vi "Running Voltmeter Average.vi"(2 "Point #":i32, 3 "Type":enum16{"DMM", "HP 34401", "Keithley 2001"}(ring), 4 "Instrument Address":refnum<visa-resource-name>) -> (0 "Stop":bool, 1 "?":dbl[](array[numeric]) format="%.4e")   [LabVIEW 2020]
doc: "This VI takes a running difference of 3 measurements of a HP34401 DMM. It assumes that the current has been reversed for the middle measurements. The value returned is the average of the 1st and 3rd measurements minus the 2nd measurement over 2.\nScott Hannahs, NHMFL - FSU, April 1995"
panel:
  out "Array":dbl[][][](array[numeric]) format="%.4e"
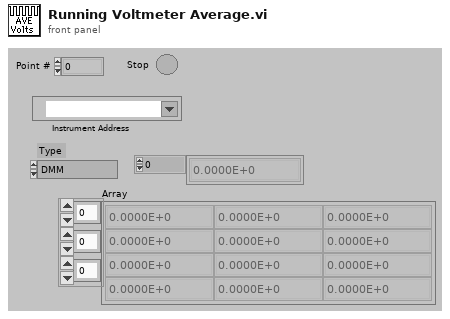
[diagram p1: front panel]
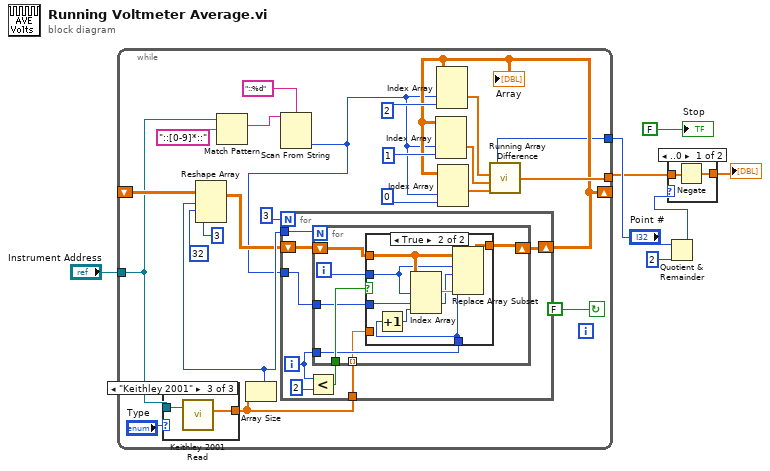
[diagram p0: block diagram]
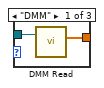
[diagram p2: hidden frame]
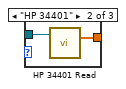
[diagram p3: hidden frame]
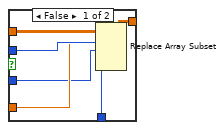
[diagram p4: hidden frame]
diagram:
  n1 = while {
    tunnel: "Point #" -> [w15]
    tunnel: "Instrument Address" -> [w8]
    tunnel: [w30] -> w4
    shift-left: _ -> [w19]
    shift-right: [w17] -> _
    stop <- FALSE continue-if-true
    n2 = case shown="\"Keithley 2001\"" "Type" {
      tunnel: w8 -> [w31 w34 w35]
      tunnel: [w32 w33 w36] -> w26
      frame "DMM" {
        n3 = call "DMM Read.vi"("Instrument Address"=w31) -> ("Measurement"=w32:dbl[])  [unwired: 1 in, 1 out]
      }
      frame "HP 34401" {
        n4 = call "HP 34401 Read.vi"("Instrument Address"=w34) -> ("Measurement"=w33:dbl[])  [unwired: 1 in, 1 out]
      }
      frame "Keithley 2001" {
        n5 = call "Keithley 2001 Read.vi"("Instrument Address"=w35) -> ("Measurement"=w36:dbl[])  [unwired: 1 in, 1 out]
      }
    }
    n6 = Match Pattern(string=w8, regular expression="::[0-9]*::") -> (match substring=w11:string)  [unwired: 1 in, 3 out]
    n7 = Array Size(array=w26) -> (size(s)=w25:i32)
    n8 = Reshape Array(w19, w25, 32, 3) -> (w18:dbl[][][])
    n9 = Scan From String(format string="::%d" ("Format String"), input string=w11) -> (output 1=w9:i32)  [unwired: 3 in, 3 out]
    n10 = for {
      N: 3 -> [_]
      tunnel: w9 -> [w39]
      tunnel: w26 -> [w44]
      tunnel: w25 -> [w40]
      shift-right: [w37] -> w17
      shift-left: w18 -> [w38]
      i -> [w43]
      n11 = Less?(x=w43, y=2) -> (x < y?=w41:bool)
      n12 = for {
        N: w40 -> [_]
        tunnel: w44 -> [w49] mode=indexing
        tunnel: w41 -> [w51]
        tunnel: w43 -> [w50]
        tunnel: w39 -> [w47]
        shift-right: [w45] -> w37
        shift-left: w38 -> [w46]
        i -> [w48]
        n13 = case shown="True" w51 {
          tunnel: w46 -> [w57 w59]
          tunnel: w50 -> [w56 w63]
          tunnel: [w55 w62] -> w45
          tunnel: w48 -> [w54 w58]
          tunnel: w49 -> [w53 _]
          tunnel: w47 -> [w52 w60]
          frame False {
            n14 = Replace Array Subset(array=w57, new element=w53, index (dim 0)=w54, index (dim 1)=w52, index (dim 2)=w56) -> (w55:dbl[][][])
          }
          frame True {
            n15 = Increment(x=w63) -> (x+1=w64:i32)
            n16 = Index Array(array=w59, index (dim 0)=w58, index (dim 1)=w60, index (dim 2)=w64) -> (element=w61:dbl)
            n17 = Replace Array Subset(array=w59, new element=w61, index (dim 0)=w58, index (dim 1)=w60, index (dim 2)=w63) -> (w62:dbl[][][])
          }
        }
      }
    }
    "Array" <- w17
    n18 = Index Array(array=w17, index (dim 1)=w9, index (dim 2)=1) -> (element=w24:dbl[])  [unwired: 1 in]
    n19 = Index Array(array=w17, index (dim 1)=w9, index (dim 2)=2) -> (element=w16:dbl[])  [unwired: 1 in]
    n20 = Index Array(array=w17, index (dim 1)=w9, index (dim 2)=0) -> (element=w23:dbl[])  [unwired: 1 in]
    n21 = call "Running Array Difference.vi"(1:w23, 2:w24, 3:w16, "Point #"=w15) -> (0:w30:dbl[])
  }
  n22 = Quotient & Remainder(x="Point #", y=2) -> (x-y*floor(x/y)=w5:i32)  [unwired: 1 out]
  n23 = case shown="..0" w5 {
    tunnel: [w65 w67] -> w2
    tunnel: w4 -> [w66 w67]
    frame ..0 {
      n24 = Negate(x=w66) -> (-x=w65:dbl[])
    }
    frame 1.. {
    }
  }
  "?" <- w2
  "Stop" <- FALSE
